vi "Status string Append--helper.vi"(10 "String":string, 11 "Data Cluster in":T1) -> (3 "Data Cluster out":T1)   [LabVIEW 2022 SP3, in "Serial-Com-Module.lvlib"]
uses:
  Serial-Com-Module.lvlib
  Module Data--cluster.ctl
  Serial Base Class/Serial Base.lvclass
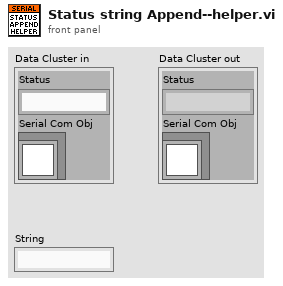
[diagram p1: front panel]
types:
  T1 = typedef "Serial-Com-Module.lvlib/Module Data--cluster.ctl" = cluster{"Status":string, "Serial Com Obj":refnum<class "Serial Base.lvclass">}
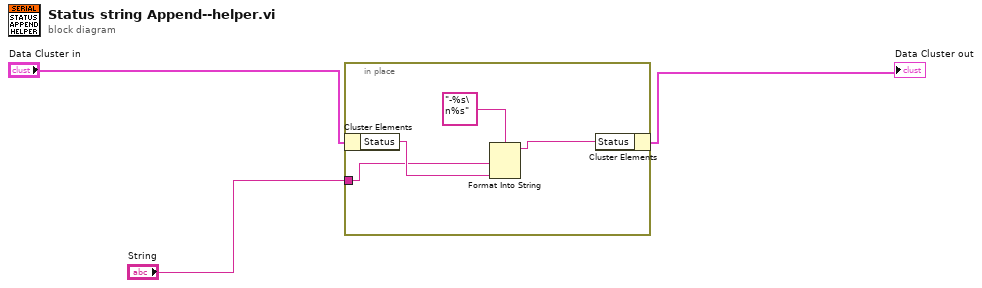
[diagram p0: block diagram]
diagram:
  n1 = in-place {
    in-place-border: "String" -> [w5]
    n2 = in-place-cluster #1("Data Cluster in") -> ("Status"=w6:string)
    n3 = Format Into String(format string="-%s\n%s", w5, w6) -> (resulting string=w4:string)  [unwired: 2 in, 1 out]
    n4 = in-place-cluster #1("Status"=w4) -> (→"Data Cluster out":T1)
  }
